vi "Teleop.vi"(10 "Match Info":T1={"Autonomous Elapsed Seconds"=0.0, "TeleOp Elapsed Seconds"=0.0, "Disabled Elapsed Seconds"=0.0, "Visited Autonomous"=FALSE, "Visited TeleOp"=FALSE, "Visited Disabled"=FALSE, "Autonomous Settings"={"Autonomous Style"=enum."Independent", "VI Refnum"=refnum}}, 11 "Call Context":T2) -> ()   [LabVIEW 2012]
doc: "This VI is called for each TeleOp packet received from the DS where the robot is not disabled. It is often used to read from the joysticks and update I/O or to update setpoints for timed control loops. It should complete and return within 20 milliseconds or it may miss DS packets."
uses:
  <vilib>/Rock Robotics/WPI/DriverStation/WPI_DriverStationDerivedRobotMode.ctl
  <vilib>/Rock Robotics/WPI/DriverStation/WPI_DriverStationMatch Info.ctl
  Robot Global Data.vi
  <vilib>/Rock Robotics/WPI/Joystick/WPI_JoystickGetSetRefNum.vi
  <vilib>/Rock Robotics/WPI/RobotDrive/WPI_RobotDriveGetSetRefNum.vi
  <vilib>/Rock Robotics/WPI/RobotDrive/WPI_RobotDriveArcadeDrive_Standard(NoSaturation).vi
  <vilib>/Rock Robotics/WPI/RobotDrive/WPI_RobotDriveArcadeDrive_ButtonSpin.vi
  <vilib>/Rock Robotics/WPI/RobotDrive/WPI_RobotDriveArcadeDrive_RatioCurve.vi
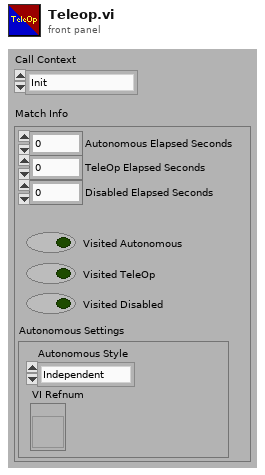
[diagram p1: front panel]
types:
  T1 = typedef "WPI_DriverStationMatch Info.ctl" = cluster{"Autonomous Elapsed Seconds":dbl, "TeleOp Elapsed Seconds":dbl, "Disabled Elapsed Seconds":dbl, "Visited Autonomous":bool, "Visited TeleOp":bool, "Visited Disabled":bool, "Autonomous Settings":cluster{"Autonomous Style":enum16{"Iterative", "Independent"}, "VI Refnum":refnum<vi>}}
  T2 = typedef "WPI_DriverStationDerivedRobotMode.ctl" = enum16{"Init", "Execute", "Stop"}
  T3 = typedef "WPI_JoystickDevRef.ctl" = cluster{"Device":T4}
  T4 = typedef "WPI_JoystickDeviceEnum.ctl" = enum16{"USB 1", "USB 2", "USB 3", "USB 4", "Kinect 1", "Kinect 2"}
  T5 = typedef "WPI_JoystickButtonState.ctl" = cluster{"Button 1":bool, "Button 2":bool, "Button 3":bool, "Button 4":bool, "Button 5":bool, "Button 6":bool, "Button 7":bool, "Button 8":bool, "Button 9":bool, "Button 10":bool, "Button 11":bool, "Button 12":bool}
  T6 = cluster{"axis 1 (x)":dbl, "axis 2 (y)":dbl, "axis 3 (throttle)":dbl, "axis 4":dbl, "axis 5":dbl, "axis 6":dbl}
  T7 = typedef "WPI_RobotDriveDevRef.ctl" = cluster{"DevStatus":errorcluster, "Motors[]":T8[], "Square Inputs":bool, "Max Output":dbl, "Isochronous":bool}
  T8 = typedef "WPI_MotorControlDeviceRef.ctl" = cluster{"DeviceStatus":errorcluster, "Type":enum16{"PWM", "CAN"}, "PWM":cluster{"Digital Module":T9, "PWM Channel":T10, "DeadBand":T11}, "CAN":cluster{"Device Number":u8, "Control Mode":T12, "Semaphore":T13, "Max Vout":dbl}, "Invert":bool, "TransformRef":T14, "InvTransformRef":T14}
  T9 = typedef "FPGA_TypedefDigitalModule.ctl" = enum16{"Digital Module 1", "Digital Module 2"}
  T10 = typedef "FPGA_DIOPWMChannel.ctl" = enum8{"PWM 1", "PWM 2", "PWM 3", "PWM 4", "PWM 5", "PWM 6", "PWM 7", "PWM 8", "PWM 9", "PWM 10", "Invalid"}
  T11 = typedef "WPI_PWMDeadband.ctl" = cluster{"Name":string, "maxPositivePwm":i32, "minPositivePwm":i32, "centerPwm":i32, "maxNegativePwm":i32, "minNegativePwm":i32, "angularRange":u16}
  T12 = typedef "WPI_CANJaguar_ControlMode.ctl" = enum8{"Percent VBus", "Current", "Speed", "Position", "Voltage"}
  T13 = typedef "Semaphore RefNum" = refnum<k1>
  T14 = typedef "WPI_PWMTransform_ConPane.ctl" = refnum<vi>
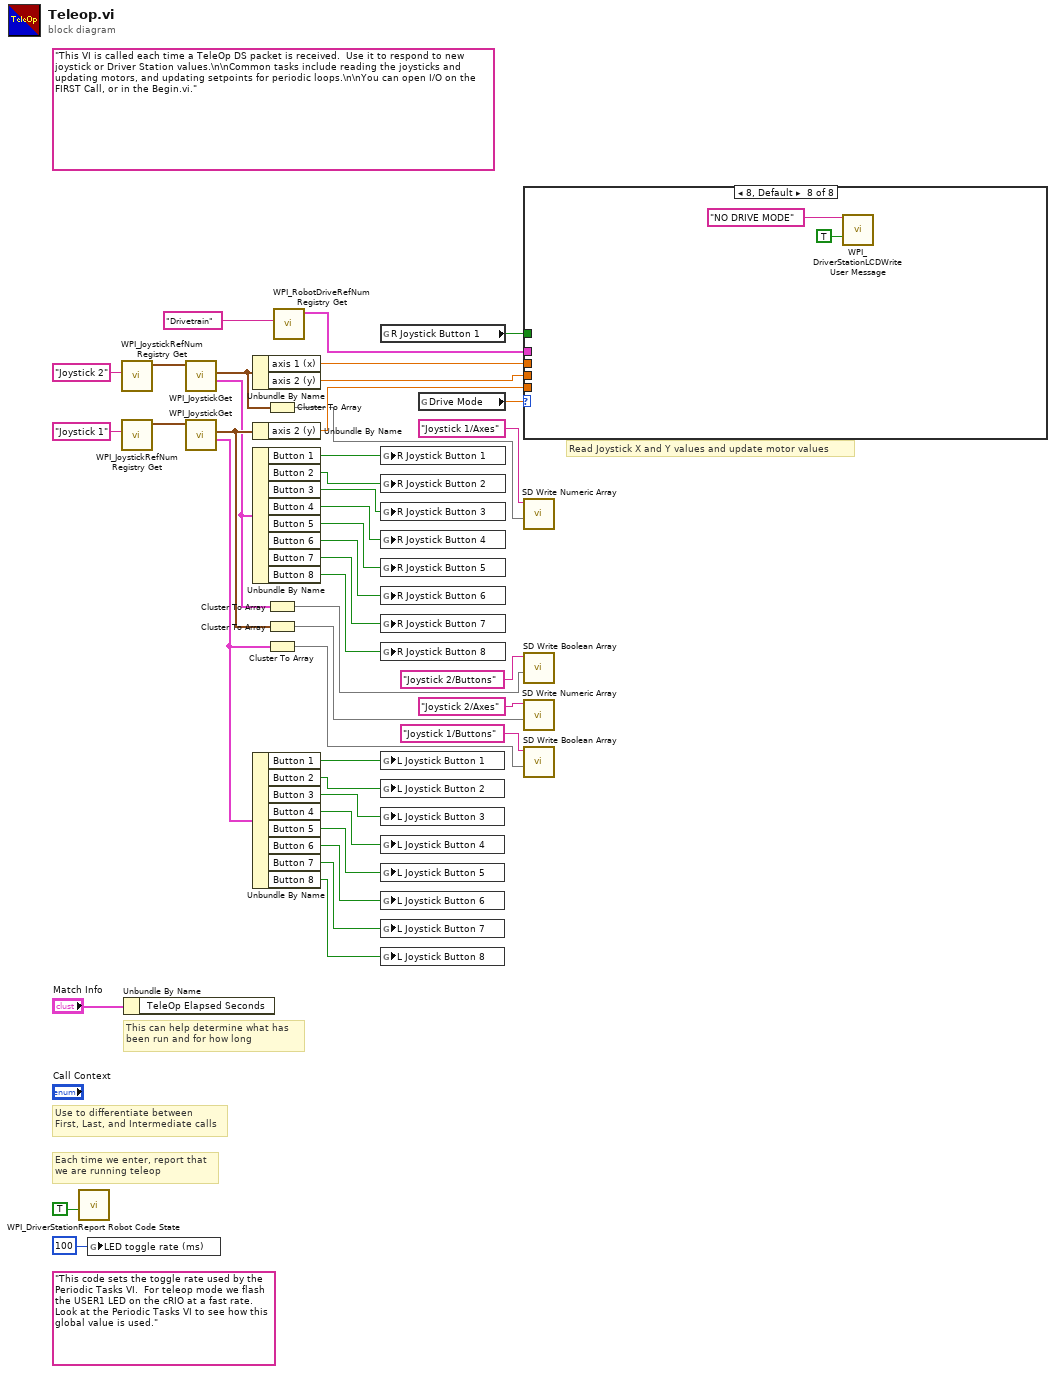
[diagram p0: block diagram]
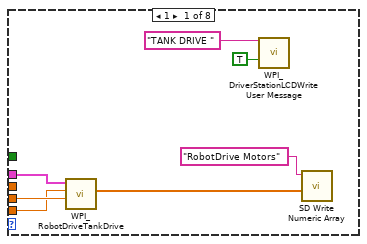
[diagram p2: hidden frame]
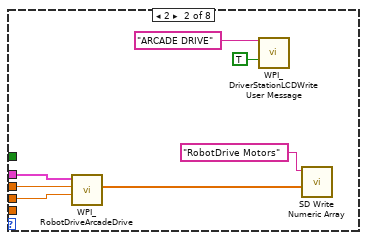
[diagram p3: hidden frame]
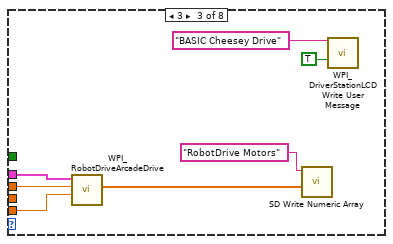
[diagram p4: hidden frame]
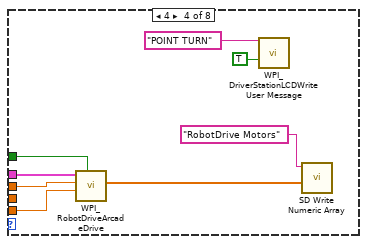
[diagram p5: hidden frame]
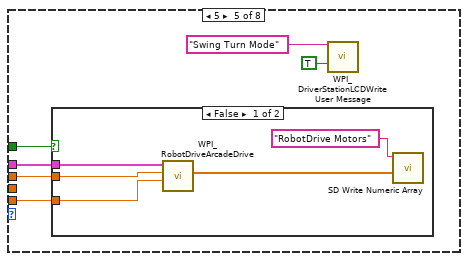
[diagram p6: hidden frame]
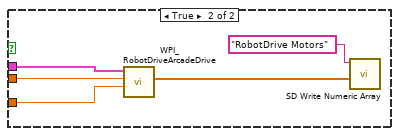
[diagram p7: hidden frame]
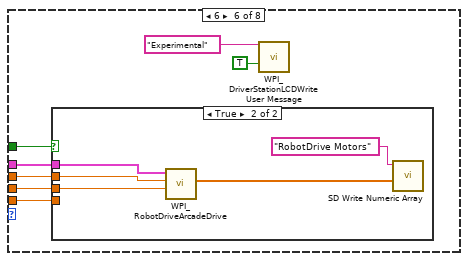
[diagram p8: hidden frame]
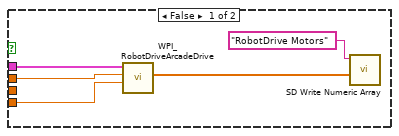
[diagram p9: hidden frame]
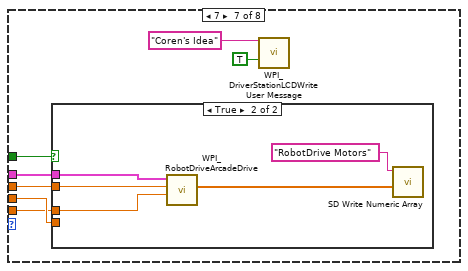
[diagram p10: hidden frame]
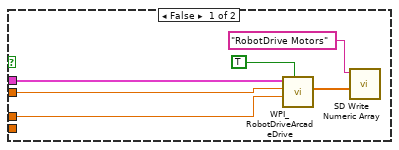
[diagram p11: hidden frame]
diagram:
  (unwired) "This code sets the toggle rate used by the Periodic Tasks VI.  For teleop mode we flash the USER1 LED on the cRIO at a fast rate.  Look at the Periodic Tasks VI to see how this global value is used."
  (unwired) "This VI is called each time a TeleOp DS packet is received.  Use it to respond to new joystick or Driver Station values.\n\nCommon tasks include reading the joysticks and updating motors, and updating setpoints for periodic loops.\n\nYou can open I/O on the FIRST Call, or in the Begin.vi."
  # "Each time we enter, report that\nwe are running teleop"
  # "Use to differentiate between\nFirst, Last, and Intermediate calls"
  # "This can help determine what has\nbeen run and for how long"
  # "Read Joystick X and Y values and update motor values"
  n1 = call <vilib>:"WPI_DriverStationReport Robot Code State.vi"("TeleOp"=TRUE ("Autonomous")) -> ()  [unwired: 10 in, 1 out]
  n2 = global write "Robot Global Data.vi" "LED toggle rate (ms)"(u32 100 ("LED ms toggle rate")) -> ()
  n3 = call <vilib>:"WPI_JoystickRefNum Registry Get.vi"("refnum name"="Joystick 2") -> ("JoystickDevRef"=w35:T3)  [unwired: 1 in, 9 out]
  n4 = call <vilib>:"WPI_JoystickRefNum Registry Get.vi"("refnum name"="Joystick 1") -> ("JoystickDevRef"=w39:T3)  [unwired: 1 in, 9 out]
  n5 = Unbundle By Name("Match Info") -> ()  [unwired: 1 out]
  n6 = call <vilib>:"WPI_JoystickGet.vi"("JoystickDevRef"=w35) -> ("Buttons"=w1:T5, "Axes"=w11:T6)  [unwired: 1 in, 4 out]
  n7 = call <vilib>:"WPI_JoystickGet.vi"("JoystickDevRef"=w39) -> ("Buttons"=w4:T5, "Axes"=w9:T6)  [unwired: 1 in, 4 out]
  n8 = Unbundle By Name(w11) -> ("axis 1 (x)"=w16:dbl, "axis 2 (y)"=w15:dbl)
  n9 = Unbundle By Name(w9) -> ("axis 2 (y)"=w14:dbl)
  n10 = Unbundle By Name(w1) -> ("Button 1"=w34:bool, "Button 2"=w33:bool, "Button 3"=w32:bool, "Button 4"=w31:bool, "Button 5"=w30:bool, "Button 6"=w29:bool, "Button 7"=w28:bool, "Button 8"=w27:bool)
  n11 = Unbundle By Name(w4) -> ("Button 1"=w26:bool, "Button 2"=w25:bool, "Button 3"=w24:bool, "Button 4"=w23:bool, "Button 5"=w22:bool, "Button 6"=w21:bool, "Button 7"=w20:bool, "Button 8"=w19:bool)
  n12 = Cluster To Array(cluster=w11) -> (array=w12:dbl[])
  n13 = Cluster To Array(cluster=w1) -> (array=w3:bool[])
  n14 = Cluster To Array(cluster=w9) -> (array=w10:dbl[])
  n15 = Cluster To Array(cluster=w4) -> (array=w6:bool[])
  n16 = call <vilib>:"WPI_RobotDriveRefNum Registry Get.vi"("refnum name"="Drivetrain") -> ("RobotDriveDevRef"=w17:T7)  [unwired: 1 in, 9 out]
  n17 = global read "Robot Global Data.vi" "R Joystick Button 1"() -> (w13:bool)
  n18 = global write "Robot Global Data.vi" "R Joystick Button 1"(w34) -> ()
  n19 = global write "Robot Global Data.vi" "R Joystick Button 2"(w33) -> ()
  n20 = global write "Robot Global Data.vi" "R Joystick Button 3"(w32) -> ()
  n21 = global write "Robot Global Data.vi" "R Joystick Button 4"(w31) -> ()
  n22 = global write "Robot Global Data.vi" "R Joystick Button 5"(w30) -> ()
  n23 = global write "Robot Global Data.vi" "R Joystick Button 6"(w29) -> ()
  n24 = global write "Robot Global Data.vi" "R Joystick Button 7"(w28) -> ()
  n25 = global write "Robot Global Data.vi" "R Joystick Button 8"(w27) -> ()
  n26 = global write "Robot Global Data.vi" "L Joystick Button 1"(w26) -> ()
  n27 = global write "Robot Global Data.vi" "L Joystick Button 2"(w25) -> ()
  n28 = global write "Robot Global Data.vi" "L Joystick Button 3"(w24) -> ()
  n29 = global write "Robot Global Data.vi" "L Joystick Button 4"(w23) -> ()
  n30 = global write "Robot Global Data.vi" "L Joystick Button 5"(w22) -> ()
  n31 = global write "Robot Global Data.vi" "L Joystick Button 6"(w21) -> ()
  n32 = global write "Robot Global Data.vi" "L Joystick Button 7"(w20) -> ()
  n33 = global write "Robot Global Data.vi" "L Joystick Button 8"(w19) -> ()
  n34 = global read "Robot Global Data.vi" "Drive Mode"() -> (w18:dbl)
  n35 = case shown="8, Default" w18 {
    tunnel: w17 -> [w45 w56 w59 w67 w74 w91 w108 _]
    tunnel: w16 -> [_ w55 w61 w69 w72 w90 w107 _]
    tunnel: w15 -> [w49 w54 _ _ _ w89 w106 _]
    tunnel: w14 -> [w48 _ w60 w68 w73 w88 w105 _]
    tunnel: w13 -> [_ _ _ w66 w75 w92 w109 _]
    frame 1 {
      n36 = call <vilib>:"WPI_RobotDriveTankDrive.vi"("Right axis value"=w49, "Left axis value"=w48, "RobotDriveDevRef"=w45) -> ("Motor Values"=w43:dbl[])  [unwired: 6 in, 2 out]
      n37 = call <vilib>:"WPI_DriverStationLCDWrite User Message.vi"("line text"="TANK DRIVE ", "clear line before write (T)"=TRUE) -> ()  [unwired: 13 in, 1 out]
      n38 = call <vilib>:"SD Write Numeric Array.vi"("Numeric Array"=w43, "Name"="RobotDrive Motors") -> ()  [unwired: 8 in, 2 out]
    }
    frame 2 {
      n39 = call-poly <vilib>:"WPI_RobotDriveArcadeDrive.vi"("Y axis value"=w54, "X axis value"=w55, "RobotDriveDevRef"=w56) -> ("Motor Values"=w50:dbl[])  [unwired: 6 in, 2 out]
      n40 = call <vilib>:"WPI_DriverStationLCDWrite User Message.vi"("line text"="ARCADE DRIVE", "clear line before write (T)"=TRUE) -> ()  [unwired: 13 in, 1 out]
      n41 = call <vilib>:"SD Write Numeric Array.vi"("Numeric Array"=w50, "Name"="RobotDrive Motors") -> ()  [unwired: 8 in, 2 out]
    }
    frame 3 {
      n42 = call-poly <vilib>:"WPI_RobotDriveArcadeDrive.vi"("Y axis value"=w60, "X axis value"=w61, "RobotDriveDevRef"=w59) -> ("Motor Values"=w57:dbl[])  [unwired: 6 in, 2 out]
      n43 = call <vilib>:"SD Write Numeric Array.vi"("Numeric Array"=w57, "Name"="RobotDrive Motors") -> ()  [unwired: 8 in, 2 out]
      n44 = call <vilib>:"WPI_DriverStationLCDWrite User Message.vi"("line text"="BASIC Cheesey Drive", "clear line before write (T)"=TRUE) -> ()  [unwired: 13 in, 1 out]
    }
    frame 4 {
      n45 = call-poly <vilib>:"WPI_RobotDriveArcadeDrive.vi"("Spin?"=w66, "Y axis value"=w68, "X axis value"=w69, "RobotDriveDevRef"=w67) -> ("Motor Values"=w64:dbl[])  [unwired: 5 in, 2 out]
      n46 = call <vilib>:"WPI_DriverStationLCDWrite User Message.vi"("line text"="POINT TURN", "clear line before write (T)"=TRUE) -> ()  [unwired: 13 in, 1 out]
      n47 = call <vilib>:"SD Write Numeric Array.vi"("Numeric Array"=w64, "Name"="RobotDrive Motors") -> ()  [unwired: 8 in, 2 out]
    }
    frame 5 {
      n48 = case shown="False" w75 {
        tunnel: w74 -> [w82 w87]
        tunnel: w73 -> [w80 w86]
        tunnel: w72 -> [w81 w85]
        frame False {
          n49 = call-poly <vilib>:"WPI_RobotDriveArcadeDrive.vi"("Y axis value"=w80, "X axis value"=w81, "RobotDriveDevRef"=w82) -> ("Motor Values"=w78:dbl[])  [unwired: 6 in, 2 out]
          n50 = call <vilib>:"SD Write Numeric Array.vi"("Numeric Array"=w78, "Name"="RobotDrive Motors") -> ()  [unwired: 8 in, 2 out]
        }
        frame True {
          n51 = call-poly <vilib>:"WPI_RobotDriveArcadeDrive.vi"("Y axis value"=w86, "X axis value"=w85, "RobotDriveDevRef"=w87) -> ("Motor Values"=w83:dbl[])  [unwired: 6 in, 2 out]
          n52 = call <vilib>:"SD Write Numeric Array.vi"("Numeric Array"=w83, "Name"="RobotDrive Motors") -> ()  [unwired: 8 in, 2 out]
        }
      }
      n53 = call <vilib>:"WPI_DriverStationLCDWrite User Message.vi"("line text"="Swing Turn Mode", "clear line before write (T)"=TRUE) -> ()  [unwired: 13 in, 1 out]
    }
    frame 6 {
      n54 = case shown="True" w92 {
        tunnel: w91 -> [w98 w104]
        tunnel: w90 -> [w99 w103]
        tunnel: w89 -> [_ w102]
        tunnel: w88 -> [w97 _]
        frame False {
          n55 = call-poly <vilib>:"WPI_RobotDriveArcadeDrive.vi"("Y axis value (Speed)"=w97, "X axis value (Curve)"=w99, "RobotDriveDevRef"=w98) -> ("Motor Values"=w95:dbl[])  [unwired: 6 in, 2 out]
          n56 = call <vilib>:"SD Write Numeric Array.vi"("Numeric Array"=w95, "Name"="RobotDrive Motors") -> ()  [unwired: 8 in, 2 out]
        }
        frame True {
          n57 = call-poly <vilib>:"WPI_RobotDriveArcadeDrive.vi"("Y axis value (Speed)"=w102, "X axis value (Curve)"=w103, "RobotDriveDevRef"=w104) -> ("Motor Values"=w100:dbl[])  [unwired: 6 in, 2 out]
          n58 = call <vilib>:"SD Write Numeric Array.vi"("Numeric Array"=w100, "Name"="RobotDrive Motors") -> ()  [unwired: 8 in, 2 out]
        }
      }
      n59 = call <vilib>:"WPI_DriverStationLCDWrite User Message.vi"("line text"="Experimental", "clear line before write (T)"=TRUE) -> ()  [unwired: 13 in, 1 out]
    }
    frame 7 {
      n60 = case shown="True" w109 {
        tunnel: w108 -> [w117 w122]
        tunnel: w107 -> [w114 w120]
        tunnel: w106 -> [_ _]
        tunnel: w105 -> [w116 w121]
        frame False {
          n61 = call-poly <vilib>:"WPI_RobotDriveArcadeDrive.vi"("Spin?"=TRUE, "Y axis value"=w116, "X axis value"=w114, "RobotDriveDevRef"=w117) -> ("Motor Values"=w112:dbl[])  [unwired: 5 in, 2 out]
          n62 = call <vilib>:"SD Write Numeric Array.vi"("Numeric Array"=w112, "Name"="RobotDrive Motors") -> ()  [unwired: 8 in, 2 out]
        }
        frame True {
          n63 = call-poly <vilib>:"WPI_RobotDriveArcadeDrive.vi"("Y axis value"=w121, "X axis value"=w120, "RobotDriveDevRef"=w122) -> ("Motor Values"=w118:dbl[])  [unwired: 6 in, 2 out]
          n64 = call <vilib>:"SD Write Numeric Array.vi"("Numeric Array"=w118, "Name"="RobotDrive Motors") -> ()  [unwired: 8 in, 2 out]
        }
      }
      n65 = call <vilib>:"WPI_DriverStationLCDWrite User Message.vi"("line text"="Coren's Idea", "clear line before write (T)"=TRUE) -> ()  [unwired: 13 in, 1 out]
    }
    frame 8, Default {
      n66 = call <vilib>:"WPI_DriverStationLCDWrite User Message.vi"("line text"="NO DRIVE MODE", "clear line before write (T)"=TRUE) -> ()  [unwired: 13 in, 1 out]
    }
  }
  n67 = call <vilib>:"SD Write Numeric Array.vi"("Numeric Array"=w12, "Name"="Joystick 1/Axes") -> ()  [unwired: 8 in, 2 out]
  n68 = call <vilib>:"SD Write Boolean Array.vi"("Boolean Array"=w3, "Name"="Joystick 2/Buttons") -> ()  [unwired: 8 in, 2 out]
  n69 = call <vilib>:"SD Write Numeric Array.vi"("Numeric Array"=w10, "Name"="Joystick 2/Axes") -> ()  [unwired: 8 in, 2 out]
  n70 = call <vilib>:"SD Write Boolean Array.vi"("Boolean Array"=w6, "Name"="Joystick 1/Buttons") -> ()  [unwired: 8 in, 2 out]
